vi "Part 2.vi"(11 "Input":string) -> (3 "Output":i64)   [LabVIEW 2021]
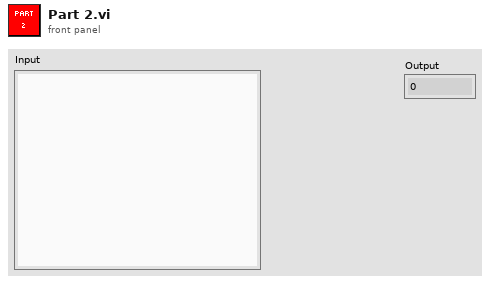
[diagram p1: front panel]
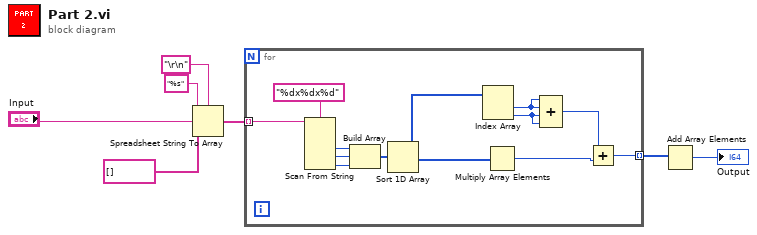
[diagram p0: block diagram]
diagram:
  n1 = Spreadsheet String To Array(delimiter (Tab)="\r\n", format string="%s", spreadsheet string="Input", array type (2D Dbl)=string[] []) -> (array=w4:string[])
  n2 = for {
    tunnel: w4 -> [w19] mode=indexing
    tunnel: [w13] -> w3 mode=indexing
    n3 = Scan From String(format string="%dx%dx%d", input string=w19) -> (output 1=w17:i32, output 2=w16:i32, output 3=w15:i32)  [unwired: 5 in, 3 out]
    n4 = Build Array(w17, w16, w15) -> (w14:i32[])
    n5 = Sort 1D Array(array=w14) -> (sorted array=w9:i32[])
    n6 = Index Array(array=w9) -> (element #1=w11:i32, element #2=w10:i32)  [unwired: 2 in]
    n7 = Multiply Array Elements(1:w9) -> (0:w12:i32)
    n8 = Compound Arithmetic op=ADD(w11, w11, w10, w10) -> (w8:i32)
    n9 = Add(x=w8, y=w12) -> (x+y=w13:i32)
  }
  n10 = Add Array Elements(numeric array=w3) -> (sum=→"Output":i32)
